vi "GetStringFeatureValue.vi"(9 "pFeatureName":string, 10 "handle":i64, 11 "error in (no error)":errorcluster) -> (1 "pStringValue":string, 2 "return type":i32, 3 "error out":errorcluster)   [LabVIEW 2016]
uses:
  MVSDKmd.dll
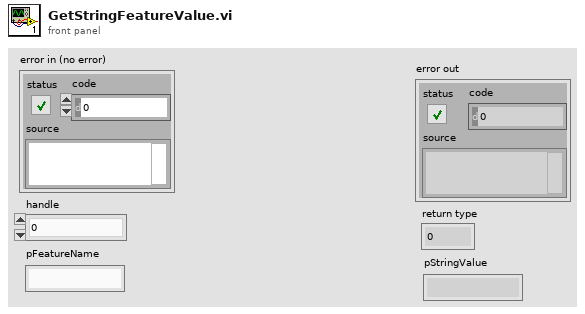
[diagram p1: front panel]
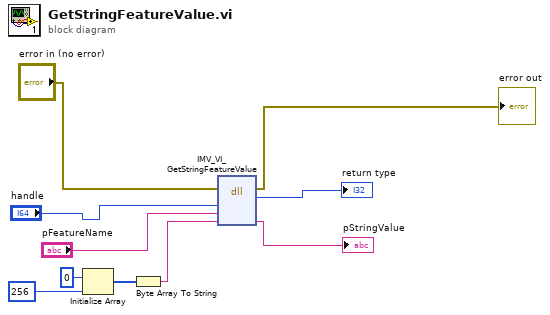
[diagram p0: block diagram]
diagram:
  n1 = Initialize Array(u8 0 ("element"), 256 ("dimension size")) -> (w4:u8[])
  n2 = Byte Array To String(unsigned byte array=w4) -> (string=w3:string)
  n3 = dll-call lib="MVSDKmd.dll" fn="IMV_VI_GetStringFeatureValue"(error in="error in (no error)", "handle"="handle", "pFeatureName"="pFeatureName", "pStringValue"=w3) -> (error out=→"error out":errorcluster, "return type"=→"return type":i32, "pStringValue"=→"pStringValue":string)  [unwired: 4 in, 1 out]
